vi "Get Category.vi"(8 "error in (no error)":errorcluster, 11 "BuckBoost editor node in":refnum<class "BuckBoost editor node.lvclass">) -> (0 "error out":errorcluster, 2 "Category":string, 3 "BuckBoost editor node out":refnum<class "BuckBoost editor node.lvclass">)   [LabVIEW 2017, in "BuckBoost editor node.lvclass"]
uses:
  BuckBoost editor node.lvclass
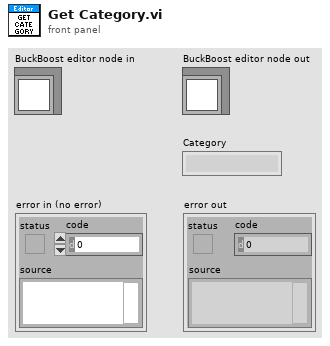
[diagram p1: front panel]
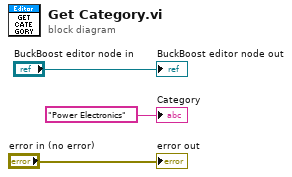
[diagram p0: block diagram]
diagram:
  "error out" <- "error in (no error)"
  "BuckBoost editor node out" <- "BuckBoost editor node in"
  "Category" <- "Power Electronics" ("Category")
